vi "UartTest.vi"() -> ()   [LabVIEW 2019]
uses:
  <vilib>/Platform/TimedLoop/XDataNode/timing_clust.ctl
  <vilib>/Platform/TimedLoop/XDataNode/nitl_modes.ctl
  <vilib>/Platform/TimedLoop/XDataNode/wakeup.ctl
  <vilib>/myRIO/Instrument Drivers/Onboard IO/UART/typedef/VISA Configuration.ctl
  <vilib>/Instr/_visa.llb/VISA Configure Serial Port (Instr).vi
  <vilib>/platform/TimedLoop/XDataNode/XDataNode.xnode
  <vilib>/myRIO/Express VI/Onboard IO/UART/UART Express VI.xnode
  <vilib>/myRIO/Instrument Drivers/Onboard IO/UART/UART.lvlib
  <vilib>/Platform/TimedLoop/XDataNode/XDNodeRunTimeDep.lvlib
panel:
  in  "RPM":u32
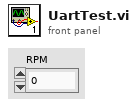
[diagram p1: front panel]
types:
  T1 = typedef "XDNodeRunTimeDep.lvlib/timing_clust.ctl" = cluster{"Expected End [f-1]":u64, "Actual End [f-1]":u64, "Finished Late? [f-1]":bool, "Expected End [i-1]":u64, "Actual End [i-1]":u64, "Finished Late? [i-1]":bool, "Expected Start [i]":u64, "Actual Start [i]":u64, "Expected Start [f]":u64, "Actual Start [f]":u64, "Source Name":string, "Structure Name":string, "Period":i64, "Deadline":i64, "Offset":i64, "Start":i64, "Priority":i32, "Timeout":i32, "Mode":T2, "Wakeup Reason":T3, "Error":errorcluster, "Source Type":string, "Secondary Source Type":string, "Global End Time":u64, "Global Start Time":u64, "Frame Duration":u64, "Iteration Duration":u64, "Assigned CPU":i32, "I/O Scan Engine Mode":u32}
  T2 = typedef "XDNodeRunTimeDep.lvlib/nitl_modes.ctl" = enum32{"No Change", "Process missed periods, maintain original phase", "Discard missed periods, maintain original phase", "Process missed periods, ignore original phase", "Discard missed periods, ignore original phase"}
  T3 = typedef "XDNodeRunTimeDep.lvlib/wakeup.ctl" = enum32{"Normal", "Aborted", "Asynchronous wakeup", "Timing source error", "Timed loop error", "Timeout"}
  T4 = typedef "UART.lvlib/VISA Configuration.ctl" = cluster{"baud rate (9600)":u32, "data bits (8)":u16, "parity (0:none)":enum16{"None", "Odd", "Even", "Mark", "Space"}, "stop bits (10: 1 bit)":u16, "flow control (0:none)":u16, "termination char\n(0xA = '\\n' = LF) ":u8, "Enable Termination\nChar (T)":bool, "timeout (10sec)":u32}
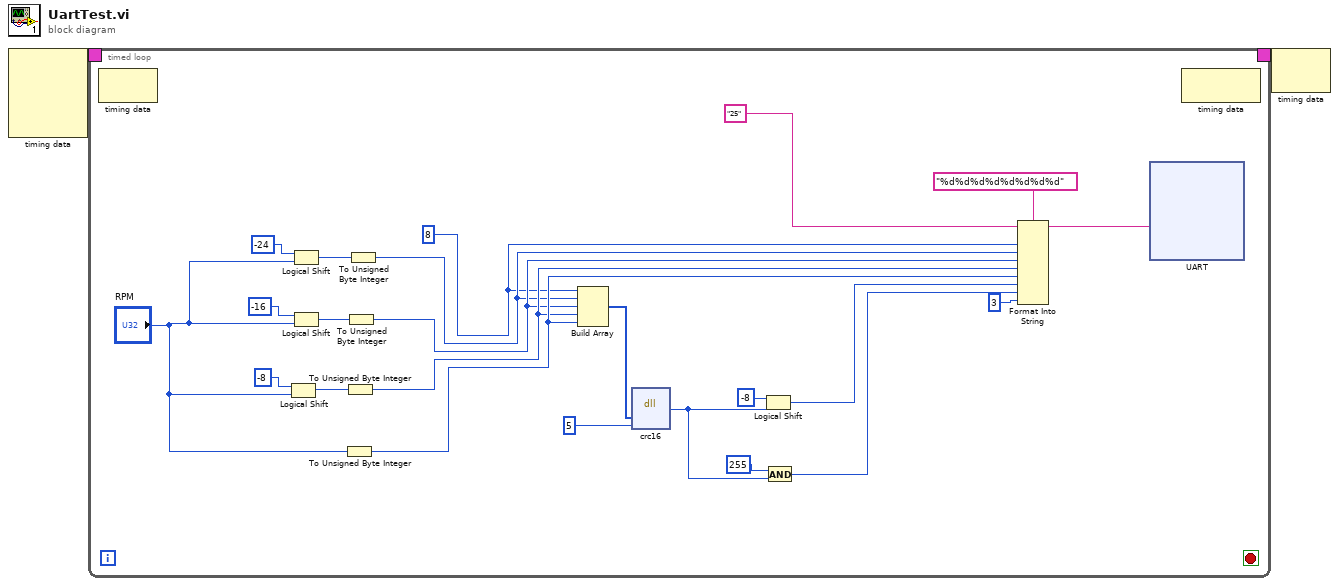
[diagram p0: block diagram]
diagram:
  n1 = node-c288() -> (w2:T1)  [unwired: 4 in]
  n2 = timed-loop {
    timing: w2 -> [_]
    timing-out: [_] -> w1
    stop <- _ stop-if-true
    w4 = 8
    n3 = node-c288() -> ()  [unwired: 1 in, 1 out]
    n4 = Logical Shift(y=i16 -8, x="RPM") -> (x << y=w20:u32)
    n5 = Logical Shift(y=i16 -24, x="RPM") -> (x << y=w24:u32)
    n6 = Logical Shift(y=i16 -16, x="RPM") -> (x << y=w21:u32)
    n7 = To Unsigned Byte Integer(number="RPM") -> (unsigned 8bit integer=w8:u8)
    n8 = To Unsigned Byte Integer(number=w20) -> (unsigned 8bit integer=w7:u8)
    n9 = To Unsigned Byte Integer(number=w21) -> (unsigned 8bit integer=w6:u8)
    n10 = To Unsigned Byte Integer(number=w24) -> (unsigned 8bit integer=w5:u8)
    n11 = Build Array(w4, w5, w6, w7, w8) -> (w18:i32[])
    n12 = dll-call lib="?" fn="crc16"("buf"=w18, "len"=5) -> ("return type"=w13:u8)  [unwired: 5 in, 2 out]
    n13 = Logical Shift(y=i16 -8, x=w13) -> (x << y=w9:u8)
    n14 = And(x=u8 255, y=w13) -> (x .and. y?=w10:u8)
    n15 = Format Into String(format string="%d%d%d%d%d%d%d%d", initial string="25", w4, w5, w6, w7, w8, w9, w10, u8 3 ("input 8")) -> (resulting string=w3:string)  [unwired: 1 in, 1 out]
    n16 = xnode "UART"("Characters to Write"=w3) -> ()  [unwired: 1 in, 2 out]
    n17 = node-c288() -> ()  [unwired: 1 in, 1 out]
  }
  n18 = node-c288(w1) -> ()  [unwired: 1 out]
